vi "Load Maze Gen.vi"(8 "error in (no error)":errorcluster, 11 "Maze Level":string) -> (0 "error out":errorcluster, 3 "MazeGen":refnum<class "MazeGen.lvclass">)   [LabVIEW 2020, in "Maze.lvlib" / "MazeGen.lvclass"]
doc: "Loads the PPL that contains the logic for generating the specific maze level. <b>Basic</b> is built into the MazeGen class but other algorithms are loaded dynamically from disk to support being distributed after the start of the challenge.\n\n<b>Errors</b>\n\n<b>-124100</b> is thrown if the specific algorithm (PPL) was not found or able to be loaded."
uses:
  MazeGen.lvclass
  <vilib>/Utility/LVLibp/NI_PackedLibraryUtility.lvlib
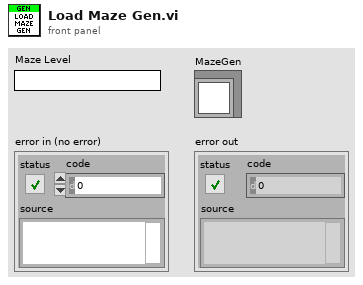
[diagram p1: front panel]
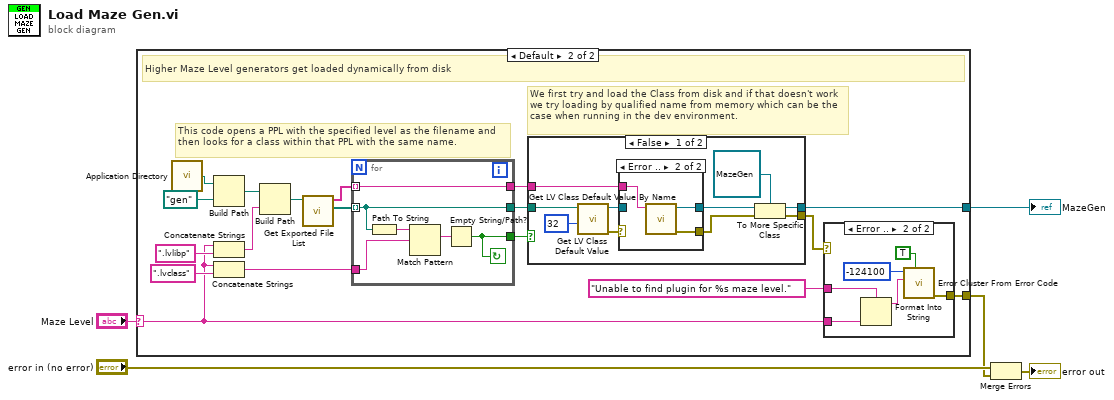
[diagram p0: block diagram]
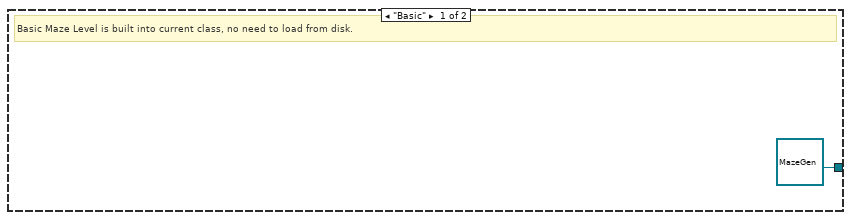
[diagram p2: hidden frame]
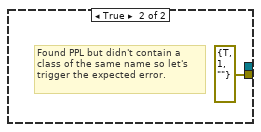
[diagram p5: hidden frame]
diagram:
  n1 = case shown="Default" "Maze Level" {
    selector: "Maze Level" -> [_ w7]
    tunnel: [refnum<class "MazeGen.lvclass"> refnum ("Maze.lvlib:MazeGen.lvclass") w11] -> w4
    tunnel: [_ w8] -> w1
    frame "Basic" {
      # "Basic Maze Level is built into current class, no need to load from disk."
    }
    frame Default {
      # "We first try and load the Class from disk and if that doesn't work we try loading by qualified name from memory which can be the case when running in the dev environment."
      # "This code opens a PPL with the specified level as the filename and then looks for a class within that PPL with the same name."
      # "Higher Maze Level generators get loaded dynamically from disk"
      n2 = call <vilib>:"Application Directory.vi"() -> ("Application Directory"=w23:path)
      n3 = Build Path(base path=w23, name or relative path=path "gen") -> (appended path=w21:path)
      n4 = Concatenate Strings(w7, ".lvlibp" ("string")) -> (w19:string)
      n5 = Concatenate Strings(w7, ".lvclass" ("string")) -> (w16:string)
      n6 = Build Path(base path=w21, name or relative path=w19) -> (appended path=w18:path)
      n7 = call <vilib>:"Get Exported File List.vi"("packed library path"=w18) -> ("paths"=w17:path[], "qualified names"=w13:string[])  [unwired: 8 in, 1 out]
      n8 = for {
        tunnel: w17 -> [w51] mode=indexing
        tunnel: [w51] -> w14
        tunnel: w16 -> [w49]
        tunnel: [w47] -> w15
        tunnel: w13 -> [w46] mode=indexing
        tunnel: [w46] -> w12
        stop <- w47 continue-if-true
        n9 = Path To String(path=w51) -> (string=w50:string)
        n10 = Match Pattern(string=w50, regular expression=w49) -> (match substring=w48:string)  [unwired: 1 in, 3 out]
        n11 = Empty String/Path?(string/path=w48) -> (empty?=w47:bool)
      }
      n12 = case shown="False" w15 {
        tunnel: w14 -> [w40 _]
        tunnel: w12 -> [w37 _]
        tunnel: [w33 _] -> w11
        tunnel: [w31 errorcluster {"status"=TRUE, "code"=1, "source"=""} ("error out")] -> w9
        frame False {
          n13 = call <vilib>:"Get LV Class Default Value.vi"("options"=u32 32, "class path"=w40) -> ("error out"=w38:errorcluster, "object"=w36:refnum<class>)  [unwired: 8 in]
          n14 = case shown="Error .." w38 {
            tunnel: w37 -> [_ w44]
            tunnel: w36 -> [w41 _]
            tunnel: [w41 w43] -> w35
            tunnel: [_ w42] -> w32
            frame No Error {
            }
            frame Error {
              n15 = call <vilib>:"Get LV Class Default Value By Name.vi"("class name"=w44) -> ("error out"=w42:errorcluster, "object"=w43:refnum<class>)  [unwired: 9 in]
            }
          }
          n16 = To More Specific Class(target class=refnum<class "MazeGen.lvclass"> refnum ("Maze.lvlib:MazeGen.lvclass"), reference=w35, error in=w32) -> (specific class reference=w33:refnum<class "MazeGen.lvclass">, error out=w31:errorcluster)
        }
        frame True {
          # "Found PPL but didn't contain a class of the same name so let's trigger the expected error."
        }
      }
      n17 = case shown="Error .." w9 {
        tunnel: "Unable to find plugin for %s maze level." -> [_ w27]
        tunnel: [_ w26] -> w8
        tunnel: w7 -> [_ w25]
        frame No Error {
        }
        frame Error {
          n18 = Format Into String(format string=w27, w25) -> (resulting string=w30:string)  [unwired: 2 in, 1 out]
          n19 = call <vilib>:"Error Cluster From Error Code.vi"("show call chain? (False)"=TRUE, "error message (\"\")"=w30, "error code (0)"=-124100) -> ("error out"=w26:errorcluster)  [unwired: 6 in]
        }
      }
    }
  }
  "MazeGen" <- w4
  n20 = Merge Errors("error in (no error)", w1) -> (→"error out":errorcluster)
